vi "Main_CP_example.vi"() -> ()   [LabVIEW 2009]
doc: "Part of the Dock/Undock demonstration of Sub Panels. Contributed by www.entzen.com.\n\nAAL 9/09"
uses:
  TD_Child_Ref_Cluster.ctl
panel:
  in  "Reposition ALL":bool
  out "loop errors":errorcluster
  in  "Undock ALL":bool
  in  "Dock ALL":bool
  out "error out":errorcluster
  out "Child_Ref Array":T1[](array[typedef])
  # "NOTE:  Child is expected to reside in the same directory as the calling parent!"
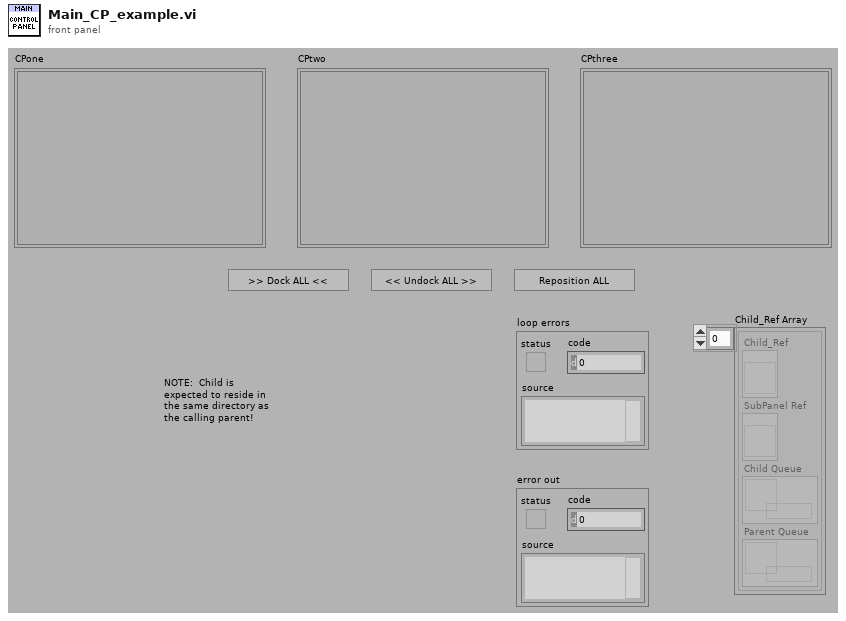
[diagram p1: front panel]
types:
  T1 = typedef "TD_Child_Ref_Cluster.ctl" = cluster{"Child_Ref":refnum<vi>, "SubPanel Ref":refnum<vi>, "Child Queue":refnum<queue>, "Parent Queue":refnum<queue>}
  T2 = enum16{"Left Button", "Center Button", "Right Button", "Window Close"}
  T3 = cluster{"Control Name":string, "type string":i16[], "data string":string}
  T4 = cluster{refnum<vi>, "CPthree":refnum<vi>, "queue out":refnum<queue>, "queue out":refnum<queue>}
  T5 = cluster{"Control Name":string, "type string":i16[], "data string":string}[]
  T6 = typedef "LVPositionTypeDef.ctl" = cluster{"Left":i32, "Top":i32}
  T7 = typedef "LVRectTypeDef.ctl" = cluster{"left":i16, "top":i16, "right":i16, "bottom":i16}
  T8 = cluster{"left":i16, "top":i16, "right":i16, "bottom":i16}
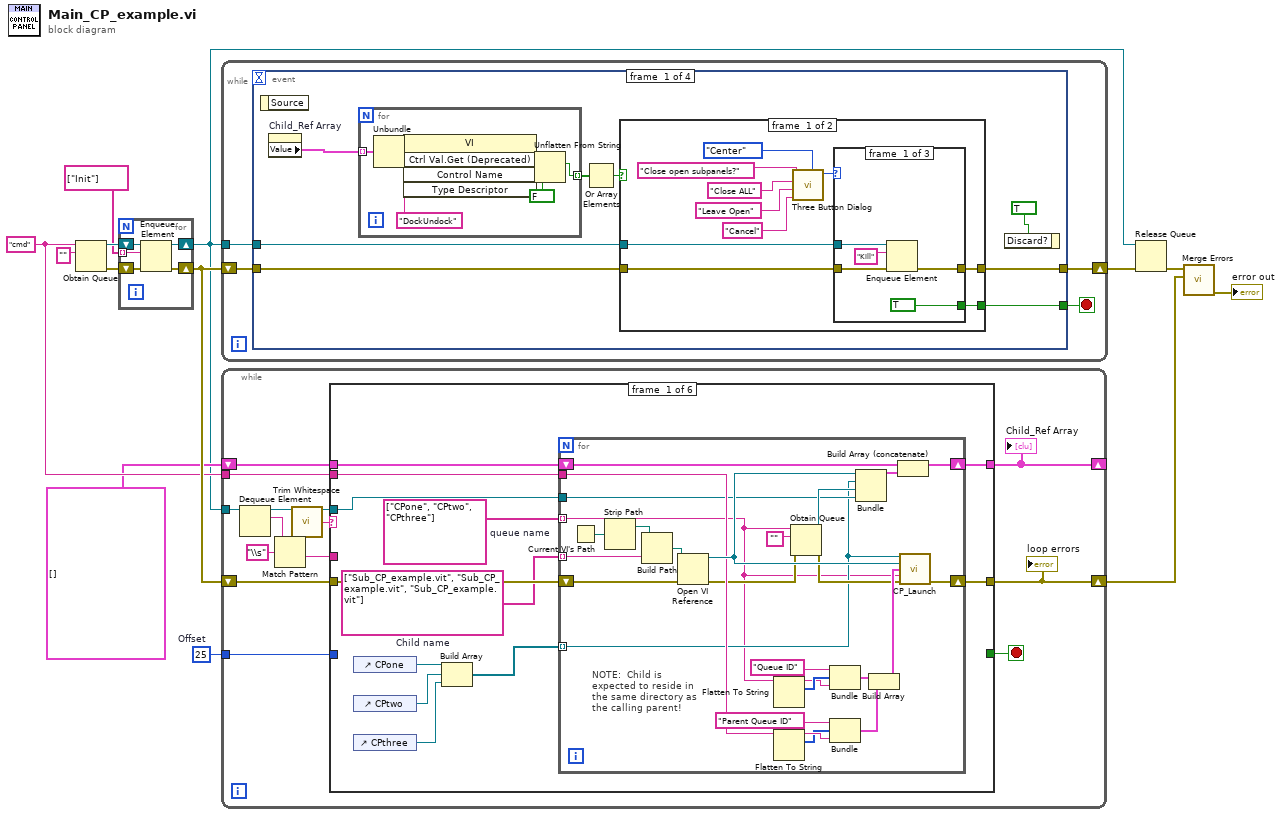
[diagram p0: block diagram]
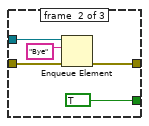
[diagram p2: hidden frame]
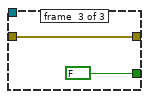
[diagram p3: hidden frame]
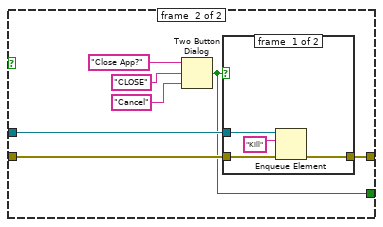
[diagram p4: hidden frame]
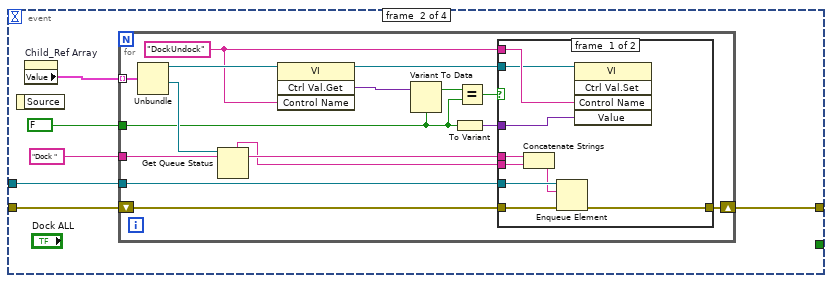
[diagram p6: hidden frame]
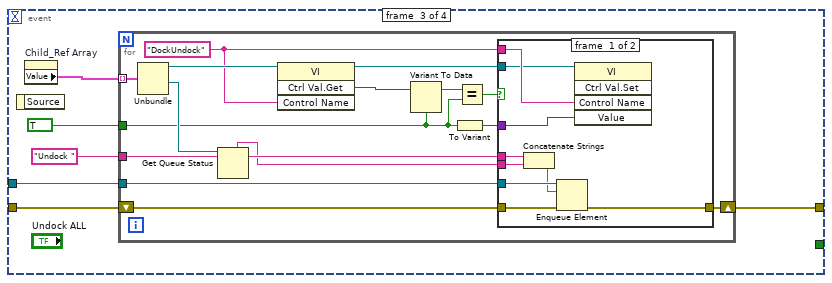
[diagram p8: hidden frame]
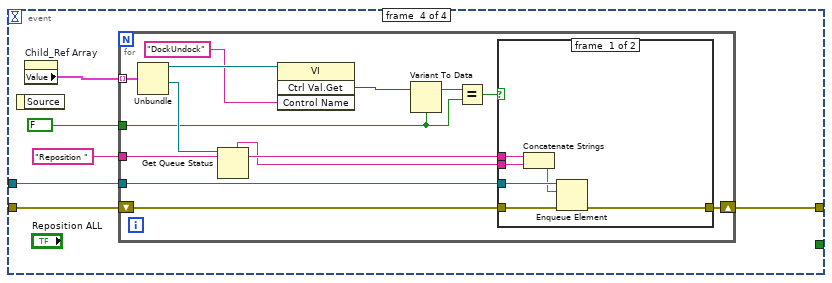
[diagram p10: hidden frame]
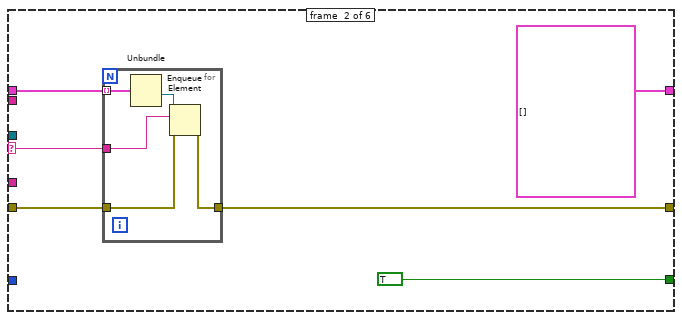
[diagram p12: hidden frame]
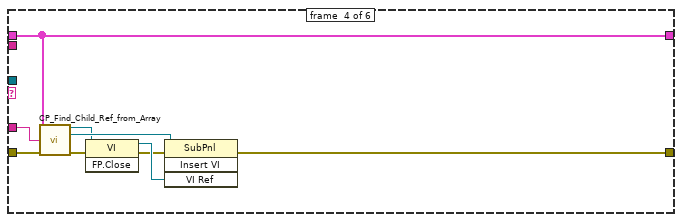
[diagram p14: hidden frame]
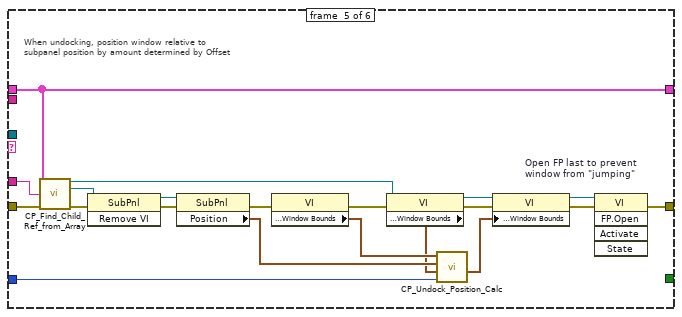
[diagram p15: hidden frame]
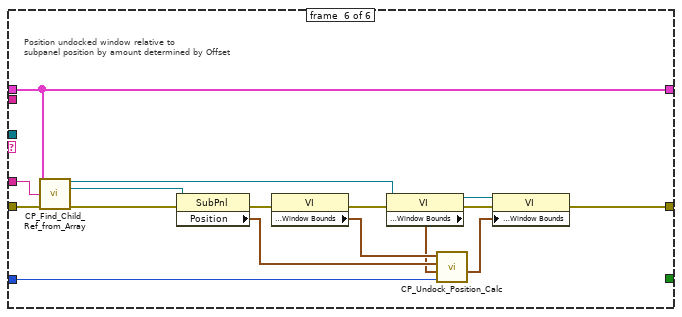
[diagram p16: hidden frame]
diagram:
  w1 = 25  # Offset
  w8 = "cmd" ("name (unnamed)")
  n1 = Obtain Queue(name (unnamed)=w8, element data type="") -> (queue out=w10:refnum<queue>, error out=w12:errorcluster)  [unwired: 3 in, 1 out]
  n2 = for {
    shift-right: [w17] -> w11
    shift-left: w12 -> [w18]
    shift-right: [w15] -> w5
    shift-left: w10 -> [w16]
    tunnel: string[] ["Init"] -> [w14] mode=indexing
    n3 = Enqueue Element(queue=w16, element=w14, error in (no error)=w18) -> (queue out=w15:refnum<queue>, error out=w17:errorcluster)  [unwired: 1 in, 1 out]
  }
  n4 = while {
    shift-right: [w21] -> w6
    shift-left: w11 -> [w22]
    tunnel: w5 -> [w20]
    stop <- w19 stop-if-true
    n5 = event shown="[3] \"Reposition ALL\": Value Change" {
      selector: _ -> [_ _ _ _]
      dyn-events: _ -> [_ _ _ _]
      timeout: _ -> [_ _ _ _]
      tunnel: w22 -> [w27 w74 w104 w134]
      tunnel: [w29 w74 w104 w134] -> w21
      tunnel: w20 -> [w30 w75 w105 w135]
      tunnel: [w23 _ _ _] -> w19
      event #0 {
        n6 = event-data() -> ()  [unwired: 1 in, 1 out]
        n7 = property on="Child_Ref Array" class="Arr (strict)"() -> ("Value"=w28:T1[])  [unwired: 2 in, 2 out]
        n8 = for {
          tunnel: w28 -> [w36] mode=indexing
          tunnel: [w31] -> w26 mode=indexing
          n9 = Unbundle(w36) -> ("Child_Ref"=w32:refnum<vi>)  [unwired: 3 out]
          n10 = invoke class="VI" method="Ctrl Val.Get (Deprecated)"(reference=w32, "Control Name"="DockUndock") -> ("Get Control Value"=w34:string)  [unwired: 3 in, 4 out]
          n11 = Unflatten From String(type=FALSE, binary string=w34) -> (value=w31:bool)  [unwired: 3 in, 2 out]
        }
        n12 = Or Array Elements(Boolean array=w26) -> (logical OR=w25:bool)
        n13 = case shown="True" w25 {
          tunnel: w27 -> [w42 w64]
          tunnel: w30 -> [w40 w63]
          tunnel: [w39 w62] -> w29
          tunnel: [w37 w59] -> w23
          frame #0 {
            n14 = call <vilib>:"Three Button Dialog.vi"("Justify Message (Left)"=enum16{"Left", "Center", "Right"}."Center", "Right Button Text (\"Cancel\")"="Cancel" ("message"), "Center Button Text (\"No\")"="Leave Open" ("message"), "Left Button Text (\"Yes\")"="Close ALL" ("message"), "message"="Close open subpanels?") -> ("Which Button?"=w41:T2)  [unwired: 6 in]
            n15 = case shown="\"Left Button\"" w41 {
              tunnel: w42 -> [w51 w56 w58]
              tunnel: w40 -> [w49 w54 _]
              tunnel: [w50 w55 w58] -> w39
              tunnel: [TRUE TRUE FALSE] -> w37
              frame #0 {
                n16 = Enqueue Element(queue=w49, element="Kill", error in (no error)=w51) -> (error out=w50:errorcluster)  [unwired: 1 in, 2 out]
              }
              frame #1 {
                n17 = Enqueue Element(queue=w54, element="Bye", error in (no error)=w56) -> (error out=w55:errorcluster)  [unwired: 1 in, 2 out]
              }
              frame #2 {
              }
            }
          }
          frame #1 {
            n18 = Two Button Dialog(message="Close App?", 1:"Cancel" ("message"), 2:"CLOSE" ("message")) -> (T button?=w59:bool)
            n19 = case shown="True" w59 {
              tunnel: w64 -> [w69 w70]
              tunnel: w63 -> [w67 _]
              tunnel: [w68 w70] -> w62
              frame #0 {
                n20 = Enqueue Element(queue=w67, element="Kill", error in (no error)=w69) -> (error out=w68:errorcluster)  [unwired: 1 in, 2 out]
              }
              frame #1 {
              }
            }
          }
        }
        n21 = event-data("Discard?"=TRUE) -> ()  [unwired: 1 in, 1 out]
      }
      event #1 {
        n22 = event-data() -> ()  [unwired: 1 in, 1 out]
        n23 = property on="Child_Ref Array" class="Arr (strict)"() -> ("Value"=w73:T1[])  [unwired: 2 in, 2 out]
        n24 = for {
          tunnel: w73 -> [w90] mode=indexing
          shift-right: [w87] -> _
          shift-left: w74 -> [w88]
          tunnel: w75 -> [w89]
          tunnel: FALSE -> [w77]
          tunnel: "Dock " ("element") -> [w86]
          w84 = "DockUndock" ("Control Name")
          n25 = Unbundle(w90) -> ("Child_Ref"=w85:refnum<vi>, "Child Queue"=w82:refnum<queue>)  [unwired: 2 out]
          n26 = Get Queue Status(queue=w82) -> (queue name=w81:string)  [unwired: 2 in, 7 out]
          n27 = invoke class="VI" method="Ctrl Val.Get"(reference=w85, "Control Name"=w84) -> (reference out=w80:refnum<vi>, "Get Control Value Variant"=w78:variant)  [unwired: 2 in, 2 out]
          n28 = Variant To Data(Variant=w78, type=w77) -> (data=w76:bool)  [unwired: 1 in, 1 out]
          n29 = To Variant(anything=w77) -> (Variant=w79:variant)
          n30 = Equal?(x=w76, y=w77) -> (x = y?=w83:bool)
          n31 = case shown="False" w83 {
            tunnel: w89 -> [w99 _]
            tunnel: w88 -> [w98 w100]
            tunnel: [w93 w100] -> w87
            tunnel: w86 -> [w96 _]
            tunnel: w84 -> [w95 _]
            tunnel: w79 -> [w94 _]
            tunnel: w81 -> [w92 _]
            tunnel: w80 -> [w91 _]
            frame #0 {
              n32 = Concatenate Strings(w96, w92) -> (w97:string)
              n33 = Enqueue Element(queue=w99, element=w97, error in (no error)=w98) -> (error out=w93:errorcluster)  [unwired: 1 in, 2 out]
              n34 = invoke class="VI" method="Ctrl Val.Set"(reference=w91, "Control Name"=w95, "Value"=w94) -> ()  [unwired: 2 in, 5 out]
            }
            frame #1 {
            }
          }
        }
      }
      event #2 {
        n35 = event-data() -> ()  [unwired: 1 in, 1 out]
        n36 = property on="Child_Ref Array" class="Arr (strict)"() -> ("Value"=w103:T1[])  [unwired: 2 in, 2 out]
        n37 = for {
          tunnel: w103 -> [w120] mode=indexing
          shift-right: [w117] -> _
          shift-left: w104 -> [w118]
          tunnel: w105 -> [w119]
          tunnel: TRUE -> [w107]
          tunnel: "Undock " ("element") -> [w116]
          w114 = "DockUndock" ("Control Name")
          n38 = Unbundle(w120) -> ("Child_Ref"=w115:refnum<vi>, "Child Queue"=w112:refnum<queue>)  [unwired: 2 out]
          n39 = Get Queue Status(queue=w112) -> (queue name=w111:string)  [unwired: 2 in, 7 out]
          n40 = invoke class="VI" method="Ctrl Val.Get"(reference=w115, "Control Name"=w114) -> (reference out=w110:refnum<vi>, "Get Control Value Variant"=w108:variant)  [unwired: 2 in, 2 out]
          n41 = Variant To Data(Variant=w108, type=w107) -> (data=w106:bool)  [unwired: 1 in, 1 out]
          n42 = To Variant(anything=w107) -> (Variant=w109:variant)
          n43 = Equal?(x=w106, y=w107) -> (x = y?=w113:bool)
          n44 = case shown="False" w113 {
            tunnel: w119 -> [w129 _]
            tunnel: w118 -> [w128 w130]
            tunnel: [w123 w130] -> w117
            tunnel: w116 -> [w126 _]
            tunnel: w114 -> [w125 _]
            tunnel: w109 -> [w124 _]
            tunnel: w111 -> [w122 _]
            tunnel: w110 -> [w121 _]
            frame #0 {
              n45 = Concatenate Strings(w126, w122) -> (w127:string)
              n46 = Enqueue Element(queue=w129, element=w127, error in (no error)=w128) -> (error out=w123:errorcluster)  [unwired: 1 in, 2 out]
              n47 = invoke class="VI" method="Ctrl Val.Set"(reference=w121, "Control Name"=w125, "Value"=w124) -> ()  [unwired: 2 in, 5 out]
            }
            frame #1 {
            }
          }
        }
      }
      event #3 {
        n48 = event-data() -> ()  [unwired: 1 in, 1 out]
        n49 = property on="Child_Ref Array" class="Arr (strict)"() -> ("Value"=w133:T1[])  [unwired: 2 in, 2 out]
        n50 = for {
          tunnel: w133 -> [w148] mode=indexing
          shift-right: [w145] -> _
          shift-left: w134 -> [w146]
          tunnel: w135 -> [w147]
          tunnel: FALSE -> [w137]
          tunnel: "Reposition " ("element") -> [w144]
          n51 = Unbundle(w148) -> ("Child_Ref"=w143:refnum<vi>, "Child Queue"=w140:refnum<queue>)  [unwired: 2 out]
          n52 = Get Queue Status(queue=w140) -> (queue name=w139:string)  [unwired: 2 in, 7 out]
          n53 = invoke class="VI" method="Ctrl Val.Get"(reference=w143, "Control Name"="DockUndock") -> ("Get Control Value Variant"=w138:variant)  [unwired: 2 in, 3 out]
          n54 = Variant To Data(Variant=w138, type=w137) -> (data=w136:bool)  [unwired: 1 in, 1 out]
          n55 = Equal?(x=w136, y=w137) -> (x = y?=w141:bool)
          n56 = case shown="False" w141 {
            tunnel: w147 -> [w154 _]
            tunnel: w146 -> [w153 w155]
            tunnel: [w150 w155] -> w145
            tunnel: w144 -> [w151 _]
            tunnel: w139 -> [w149 _]
            frame #0 {
              n57 = Concatenate Strings(w151, w149) -> (w152:string)
              n58 = Enqueue Element(queue=w154, element=w152, error in (no error)=w153) -> (error out=w150:errorcluster)  [unwired: 1 in, 2 out]
            }
            frame #1 {
            }
          }
        }
      }
    }
  }
  n59 = while {
    shift-right: [w157] -> w3
    shift-left: w11 -> [w161]
    tunnel: w5 -> [w168]
    shift-right: [w158] -> _
    shift-left: T1[] [] ("Child_Ref Array") -> [w160]
    tunnel: w8 -> [w159]
    tunnel: w1 -> [w156]
    stop <- w169 stop-if-true
    n60 = Dequeue Element(queue=w168) -> (queue out=w167:refnum<queue>, element=w164:string)  [unwired: 2 in, 2 out]
    n61 = Match Pattern(string=w164, regular expression="\\s") -> (before substring=w165:string, after substring=w162:string)  [unwired: 1 in, 2 out]
    n62 = call <vilib>:"Trim Whitespace.vi"("string"=w165) -> ("trimmed string"=w163:string)  [unwired: 1 in]
    n63 = case shown="Default" w163 {
      selector: w163 -> [_ w211 _ _ _ _]
      tunnel: [_ TRUE _ _ _ _] -> w169
      tunnel: w161 -> [w179 w214 w221 w229 w250 w266]
      tunnel: [w178 w209 w221 w230 w237 w254] -> w157
      tunnel: w167 -> [w176 _ _ _ _ _]
      tunnel: w162 -> [_ _ _ w228 w249 w265]
      tunnel: w160 -> [w181 w213 w220 w227 w247 w264]
      tunnel: [w180 T1[] [] ("Child_Ref Array") w220 w227 w247 w264] -> w158
      tunnel: w159 -> [w177 _ _ _ _ _]
      tunnel: w156 -> [_ _ _ _ w231 w251]
      frame #0 {
        w174 = string[] ["Sub_CP_example.vit", "Sub_CP_example.vit", "Sub_CP_example.vit"]  # Child name
        w175 = string[] ["CPone", "CPtwo", "CPthree"]  # queue name
        n64 = control-ref of="CPone"() -> (w173:refnum<vi>)
        n65 = control-ref of="CPtwo"() -> (w172:refnum<vi>)
        n66 = control-ref of="CPthree"() -> (w170:refnum<vi>)
        n67 = Build Array(w173, w172, w170) -> (w171:refnum<vi>[])
        n68 = for {
          tunnel: w174 -> [w202] mode=indexing
          tunnel: w177 -> [w189]
          tunnel: w175 -> [w182] mode=indexing
          tunnel: w176 -> [w184]
          shift-right: [w204] -> w180
          shift-left: w181 -> [w205]
          shift-right: [w194] -> w178
          shift-left: w179 -> [w195]
          tunnel: w171 -> [w183] mode=indexing
          # "NOTE:  Child is expected to reside in the same directory as the calling parent!"
          n69 = Current VI's Path() -> (path=w206:path)
          n70 = Strip Path(path=w206) -> (stripped path=w207:path)  [unwired: 1 out]
          n71 = Build Path(base path=w207, name or relative path=w202) -> (appended path=w208:path)
          n72 = Open VI Reference(vi path=w208, error in (no error)=w195) -> (vi reference=w196:refnum<vi>, error out=w188:errorcluster)  [unwired: 4 in]
          n73 = Flatten To String(anything=w182) -> (data string=w199:string, type string=w200:i16[])  [unwired: 3 in, 1 out]
          n74 = Flatten To String(anything=w189) -> (data string=w193:string, type string=w192:i16[])  [unwired: 3 in, 1 out]
          n75 = Obtain Queue(name (unnamed)=w182, element data type="", error in (no error)=w188) -> (queue out=w185:refnum<queue>, error out=w187:errorcluster)  [unwired: 2 in, 1 out]
          n76 = Bundle("Control Name"="Queue ID", "type string"=w200, "data string"=w199) -> (w198:T3)  [unwired: 1 in]
          n77 = Bundle("Control Name"="Parent Queue ID", "type string"=w192, "data string"=w193) -> (w190:T3)  [unwired: 1 in]
          n78 = Bundle(w196, "CPthree"=w183, "queue out"=w185, "queue out"=w184) -> (w203:T4)  [unwired: 1 in]
          n79 = Build Array(w198, w190) -> (w197:T5)
          n80 = Build Array (concatenate)(w205, w203) -> (w204:T1[])
          n81 = call "CP_Launch.vi"("SubPanel Ref"=w183, "vi reference"=w196, "Control Init Array"=w197, "Window Title (opt)"=w182, "error in (no error)"=w187) -> ("error out"=w194:errorcluster)  [unwired: 10 in]
        }
      }
      frame #1 {
        n82 = for {
          tunnel: w214 -> [w217]
          tunnel: w213 -> [w219] mode=indexing
          tunnel: [w216] -> w209
          tunnel: w211 -> [w218]
          n83 = Unbundle(w219) -> ("Child Queue"=w215:refnum<queue>)  [unwired: 3 out]
          n84 = Enqueue Element(queue=w215, element=w218, error in (no error)=w217) -> (error out=w216:errorcluster)  [unwired: 1 in, 2 out]
        }
      }
      frame #2 {
      }
      frame #3 {
        n85 = call "CP_Find_Child_Ref_from_Array.vi"("Child_Ref Array"=w227, "Queue ID"=w228, "error in (no error)"=w229) -> ("Child_Ref out"=w223:refnum<vi>, "SubPanel Ref"=w226:refnum<vi>, "error out"=w222:errorcluster)  [unwired: 7 in, 3 out]
        n86 = invoke class="VI" method="FP.Close"(reference=w223, error in=w222) -> (reference out=w225:refnum<vi>, error out=w224:errorcluster)  [unwired: 1 in, 1 out]
        n87 = invoke on="Invoke Node" class="SubPnl" method="Insert VI"(reference=w226, error in=w224, "VI Ref"=w225) -> (error out=w230:errorcluster)  [unwired: 1 in, 3 out]
      }
      frame #4 {
        # "When undocking, position window relative to\nsubpanel position by amount determined by Offset"
        n88 = call "CP_Find_Child_Ref_from_Array.vi"("Child_Ref Array"=w247, "Queue ID"=w249, "error in (no error)"=w250) -> ("Child_Ref out"=w240:refnum<vi>, "SubPanel Ref"=w246:refnum<vi>, "error out"=w248:errorcluster)  [unwired: 7 in, 3 out]
        n89 = invoke on="Invoke Node" class="SubPnl" method="Remove VI"(reference=w246, error in=w248) -> (reference out=w245:refnum<vi>, error out=w244:errorcluster)  [unwired: 1 in, 1 out]
        n90 = property on="Property Node" class="SubPnl"(reference=w245, error in=w244) -> (error out=w243:errorcluster, "Position"=w234:T6)  [unwired: 1 out]
        n91 = property on="Property Node" class="VI"(error in=w243) -> (error out=w235:errorcluster, "Front Panel Window:Window Bounds"=w236:T7)  [unwired: 1 in, 1 out]
        n92 = property on="Property Node" class="VI"(reference=w240, error in=w235) -> (reference out=w241:refnum<vi>, error out=w242:errorcluster, "Front Panel Window:Window Bounds"=w233:T7)
        n93 = call "CP_Undock_Position_Calc.vi"("Offset"=w231, "subVI FP WinBounds In"=w233, "SubPanel Position"=w234, "Main FP WinBounds"=w236) -> ("subVI FP Window Bounds Out"=w232:T8)  [unwired: 7 in]
        n94 = property on="Property Node" class="VI"(reference=w241, error in=w242, "Front Panel Window:Window Bounds"=w232) -> (reference out=w238:refnum<vi>, error out=w239:errorcluster)
        n95 = invoke on="Open FP last to prevent\nwindow from \"jumping\"" class="VI" method="FP.Open"(reference=w238, error in=w239) -> (error out=w237:errorcluster)  [unwired: 3 in, 4 out]
      }
      frame #5 {
        # "Position undocked window relative to\nsubpanel position by amount determined by Offset"
        n96 = call "CP_Find_Child_Ref_from_Array.vi"("Child_Ref Array"=w264, "Queue ID"=w265, "error in (no error)"=w266) -> ("Child_Ref out"=w260:refnum<vi>, "SubPanel Ref"=w252:refnum<vi>, "error out"=w253:errorcluster)  [unwired: 7 in, 3 out]
        n97 = property on="Property Node" class="SubPnl"(reference=w252, error in=w253) -> (error out=w263:errorcluster, "Position"=w257:T6)  [unwired: 1 out]
        n98 = property on="Property Node" class="VI"(error in=w263) -> (error out=w258:errorcluster, "Front Panel Window:Window Bounds"=w259:T7)  [unwired: 1 in, 1 out]
        n99 = property on="Property Node" class="VI"(reference=w260, error in=w258) -> (reference out=w261:refnum<vi>, error out=w262:errorcluster, "Front Panel Window:Window Bounds"=w256:T7)
        n100 = call "CP_Undock_Position_Calc.vi"("Offset"=w251, "subVI FP WinBounds In"=w256, "SubPanel Position"=w257, "Main FP WinBounds"=w259) -> ("subVI FP Window Bounds Out"=w255:T8)  [unwired: 7 in]
        n101 = property on="Property Node" class="VI"(reference=w261, error in=w262, "Front Panel Window:Window Bounds"=w255) -> (error out=w254:errorcluster)  [unwired: 1 out]
      }
    }
    "Child_Ref Array" <- w158
    "loop errors" <- w157
  }
  n102 = Release Queue(queue=w5, error in (no error)=w6) -> (error out=w4:errorcluster)  [unwired: 1 in, 2 out]
  n103 = call <vilib>:"Merge Errors.vi"("error in 2 (no error)"=w3, "error in 1 (no error)"=w4) -> ("error out"=→"error out":errorcluster)  [unwired: 5 in]
